vi "colors.vi"   [LabVIEW 2012]
uses:
  <vilib>/addons/internet/NI_InternetTK_Core_VIs.lvlib
  <vilib>/addons/internet/NI_InternetTK_Common_VIs.lvlib
types:
  T1 = typedef "CGI Connection Info.ctl" = cluster{"name":string, "type":T2, "session":T3}
  T2 = typedef "CGI Request Type.ctl" = enum16{"cgi", ".spool first", ".spool", ".spool last"}
  T3 = typedef "HTTP Session.ctl" = refnum<k1>
  T4 = typedef "NI_FTP.lvlib/Keyed Array.ctl" = cluster{"keys":string[], "values":string[]}
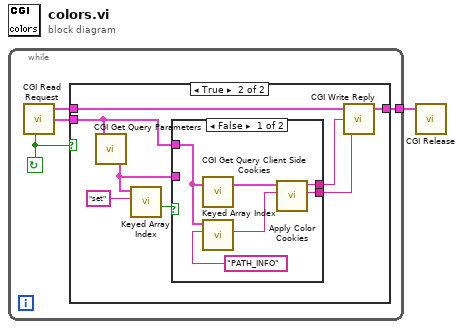
[diagram p0: block diagram]
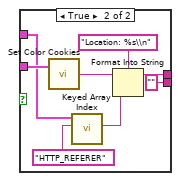
[diagram p3: hidden frame]
diagram:
  n1 = while {
    tunnel: [w4] -> w1
    stop <- w3 continue-if-true
    n2 = call <vilib>:"CGI Read Request.vi"() -> ("valid request?"=w3:bool, "cgi connection info"=w5:T1, "env"=w2:T4)  [unwired: 4 in, 1 out]
    n3 = case shown="True" w3 {
      tunnel: [w6 w14] -> w4
      tunnel: w5 -> [w6 w13]
      tunnel: w2 -> [_ w9]
      frame False {
      }
      frame True {
        n4 = call <vilib>:"CGI Get Query Parameters.vi"("env"=w9) -> ("query params"=w7:T4)  [unwired: 2 out]
        n5 = call <vilib>:"Keyed Array Index.vi"("key"="set", "array in"=w7) -> ("valid key"=w11:bool)  [unwired: 3 in, 2 out]
        n6 = case shown="False" w11 {
          tunnel: [w17 w25] -> w10
          tunnel: w7 -> [_ w24]
          tunnel: w9 -> [w19 w21]
          tunnel: [w16 "" ("content")] -> w8
          frame False {
            n7 = call <vilib>:"CGI Get Query Client Side Cookies.vi"("env"=w19) -> ("client cookies"=w18:T4)  [unwired: 1 in, 1 out]
            n8 = call <vilib>:"Keyed Array Index.vi"("key"="PATH_INFO", "array in"=w19) -> ("value"=w15:string)  [unwired: 3 in, 2 out]
            n9 = call "Apply Color Cookies.vi"("virtual document path"=w15, "client cookies"=w18) -> ("content"=w16:string, "header"=w17:string)  [unwired: 4 in]
          }
          frame True {
            n10 = call "Set Color Cookies.vi"("query params"=w24) -> ("Header Lines"=w23:string)  [unwired: 1 in]
            n11 = call <vilib>:"Keyed Array Index.vi"("key"="HTTP_REFERER", "array in"=w21) -> ("value"=w26:string)  [unwired: 3 in, 2 out]
            n12 = Format Into String(format string="Location: %s\\n", initial string=w23, w26) -> (resulting string=w25:string)  [unwired: 1 in, 1 out]
          }
        }
        n13 = call <vilib>:"CGI Write Reply.vi"("content"=w8, "header"=w10, "cgi connection info"=w13) -> ("cgi connection info out"=w14:T1)  [unwired: 2 in]
      }
    }
  }
  n14 = call <vilib>:"CGI Release.vi"("cgi connection info"=w1) -> ()  [unwired: 5 in]
